vi "Convert_data_variant_to_data_string.vi"(0 "datatype":T1, 5 "data in":variant, 11 "error in (no error)":errorcluster) -> (4 "String":string, 15 "error out":errorcluster)   [LabVIEW 2019, in "mmW_commands.lvlib"]
uses:
  mmW_commands.lvlib
  <vilib>/addons/_JKI.lib/Serialization/JSON/JKI JSON Serialization.lvlib
  commands/typedefs/datatypes_.ctl
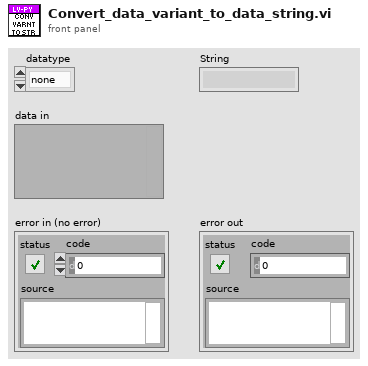
[diagram p1: front panel]
types:
  T1 = typedef "mmW_commands.lvlib/datatypes_.ctl" = enum16{"none", "string", "interleaved_I16", "interleaved_I32", "I16_array", "I32_array", "JSONstring"}
  T2 = enum16{"big-endian, network order", "native, host order", "little-endian"}
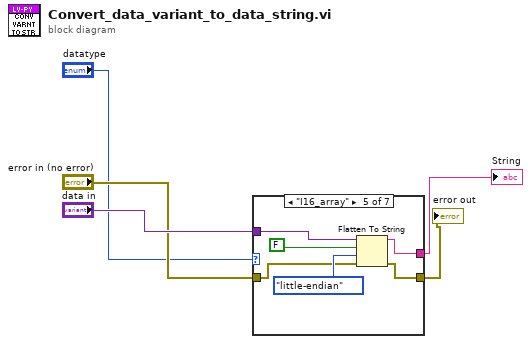
[diagram p0: block diagram]
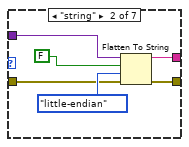
[diagram p3: hidden frame]
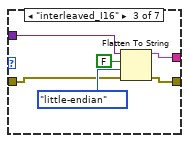
[diagram p4: hidden frame]
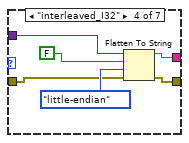
[diagram p5: hidden frame]
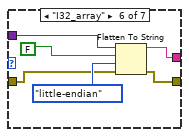
[diagram p6: hidden frame]
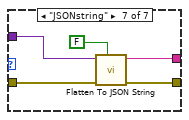
[diagram p7: hidden frame]
diagram:
  n1 = case shown="\"I16_array\"" "datatype" {
    tunnel: [w6 w10 w14 w21 w27 w32 w40] -> w5
    tunnel: [_ w9 w13 w22 w28 w31 w39] -> w4
    tunnel: "error in (no error)" -> [w6 w8 w15 w20 w26 w33 w38]
    tunnel: "data in" -> [_ w7 w17 w23 w29 w35 w37]
    frame "none", Default {
    }
    frame "string" {
      n2 = Flatten To String(anything=w7, prepend array or string size? (T)=FALSE, byte order (0:big-endian, network order)=T2."little-endian", error in (no error)=w8) -> (data string=w9:string, error out=w10:errorcluster)  [unwired: 1 out]
    }
    frame "interleaved_I16" {
      n3 = Flatten To String(anything=w17, prepend array or string size? (T)=FALSE, byte order (0:big-endian, network order)=T2."little-endian", error in (no error)=w15) -> (data string=w13:string, error out=w14:errorcluster)  [unwired: 1 out]
    }
    frame "interleaved_I32" {
      n4 = Flatten To String(anything=w23, prepend array or string size? (T)=FALSE, byte order (0:big-endian, network order)=T2."little-endian", error in (no error)=w20) -> (data string=w22:string, error out=w21:errorcluster)  [unwired: 1 out]
    }
    frame "I16_array" {
      n5 = Flatten To String(anything=w29, prepend array or string size? (T)=FALSE, byte order (0:big-endian, network order)=T2."little-endian", error in (no error)=w26) -> (data string=w28:string, error out=w27:errorcluster)  [unwired: 1 out]
    }
    frame "I32_array" {
      n6 = Flatten To String(anything=w35, prepend array or string size? (T)=FALSE, byte order (0:big-endian, network order)=T2."little-endian", error in (no error)=w33) -> (data string=w31:string, error out=w32:errorcluster)  [unwired: 1 out]
    }
    frame "JSONstring" {
      n7 = call <vilib>:"Flatten To JSON String.vi"("Multiline (T)"=FALSE, "error in (no error)"=w38, "Variant"=w37) -> ("error out"=w40:errorcluster, "JSON String"=w39:string)  [unwired: 7 in]
    }
  }
  "error out" <- w5
  "String" <- w4
